vi "Initialize Stream VI.vi"(8 "error in (no error)":errorcluster, 11 "Roda_Filtros in":refnum<class "Roda_Filtros.lvclass">) -> (0 "error out":errorcluster, 3 "Roda_Filtros out":refnum<class "Roda_Filtros.lvclass">)   [LabVIEW 2018, in "Roda_Filtros.lvclass"]
uses:
  Roda_Filtros.lvclass
  Roda_Filtros.lvclass/Roda_Filtros.ctl
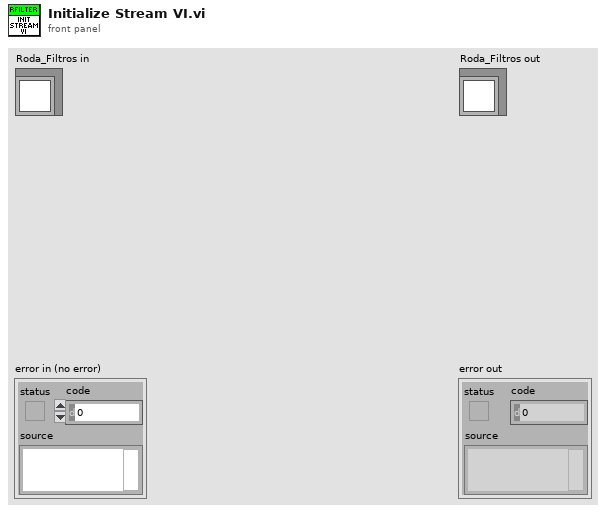
[diagram p1: front panel]
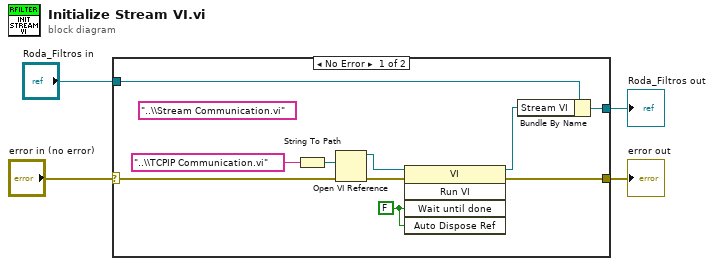
[diagram p0: block diagram]
diagram:
  n1 = case shown="No Error" "error in (no error)" {
    selector: "error in (no error)" -> [w11 w16]
    tunnel: [w10 w16] -> w3
    tunnel: [w8 w15] -> w1
    tunnel: "Roda_Filtros in" -> [w9 w15]
    frame No Error {
      (unwired) "..\\Stream Communication.vi"
      w13 = FALSE ("Wait Until Done")
      n2 = String To Path(string="..\\TCPIP Communication.vi") -> (path=w5:path)
      n3 = Open VI Reference(vi path=w5, error in (no error)=w11) -> (vi reference=w14:refnum<vi>, error out=w12:errorcluster)  [unwired: 4 in]
      n4 = invoke class="VI" method="Run VI"(reference=w14, error in=w12, "Wait until done"=w13, "Auto Dispose Ref"=w13) -> (reference out=w7:refnum<vi>, error out=w10:errorcluster)  [unwired: 1 in, 3 out]
      n5 = Bundle By Name(cluster=w9, "Stream VI"=w7) -> (w8:refnum<class "Roda_Filtros.lvclass">)
    }
    frame Error {
    }
  }
  "error out" <- w3
  "Roda_Filtros out" <- w1
